vi "Less.vi"() -> ()   [LabVIEW 2017, in "Assertions.Tests.lvlib" / "Assert Less Than or Equal To.lvlib"]
uses:
  Assert Less Than or Equal To.lvlib
  8473c714-3a53-4988-b2b2-14cc8396fd65.vi
  src/Transparent Assertions/Constraints/Logical Or/Logical Or.lvclass
  C:/Users/pasca/Projects/Home/TransparentAssertions/src/Transparent Assertions/Constraints/Binary Operator/Binary Operator.lvclass
  src/Transparent Assertions/Constraints/Is Less Than/Is Less Than.lvclass
  C:/Users/pasca/Projects/Home/TransparentAssertions/src/Transparent Assertions/Constraints/Constraint/Constraint.lvclass
  src/Transparent Assertions/Constraints/IsEqual/IsEqual.lvclass
  src/Transparent Assertions/Constraints/IsEqual/Create.vi
  src/Transparent Assertions/Constraints/Is Less Than/Create.vi
  src/Transparent Assertions/Constraints/Binary Operator/Create.vi
  src/Transparent Assertions/Assertions/Assertions.lvlib
panel:
  out "error out":errorcluster
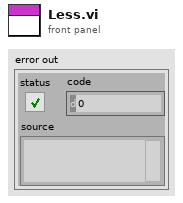
[diagram p1: front panel]
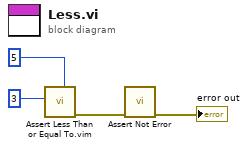
[diagram p0: block diagram]
diagram:
  n1 = call "Assert Less Than or Equal To.vim"("Expected"=5, "Actual"=3) -> ("error out"=w3:errorcluster)  [unwired: 9 in]
  n2 = call "Assert Not Error.vi"("error in (no error)"=w3) -> ("error out"=→"error out":errorcluster)  [unwired: 10 in]
